vi "fix_shared_library_paths_for_package.vi"(8 "error in":errorcluster, 11 "Package File Path":path) -> (0 "error out":errorcluster)   [LabVIEW 2020]
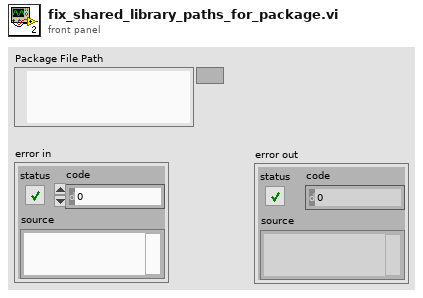
[diagram p1: front panel]
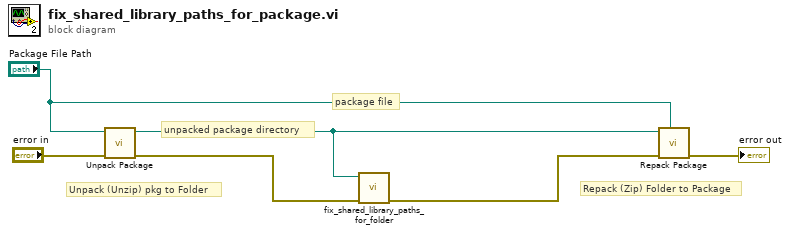
[diagram p0: block diagram]
diagram:
  # "Repack (Zip) Folder to Package"
  # "Unpack (Unzip) pkg to Folder"
  # "package file"
  # "unpacked package directory"
  n1 = call "Unpack Package.vi"("error in (no error)"="error in", "Package File"="Package File Path") -> ("error out"=w4:errorcluster, "Unpacked Package Directory"=w5:path)  [unwired: 7 in, 1 out]
  n2 = call "fix_shared_library_paths_for_folder.vi"("error in"=w4, "Folder of VIs"=w5) -> ("error out"=w3:errorcluster)  [unwired: 9 in]
  n3 = call "Repack Package.vi"("Package File (\"\": use name of directory to repack)"="Package File Path", "error in (no error)"=w3, "Directory to repack"=w5) -> ("error out"=→"error out":errorcluster)  [unwired: 8 in]
